vi "ReadDataByIdentifier.vi"(5 "LogSuspend":bool, 8 "error in":errorcluster, 10 "DID":string="02 02", 11 "UdsHandleIn":T1={"LogPath"=path "", "LogEnabled"=FALSE, "isOpen"=FALSE, "LogContent"="", "Adapter"="CAN0", "MCanHandle"={"MCanAdapter"=refnum}, "TransmittId"=0, "ReceiveId"=0}) -> (0 "error out":errorcluster, 2 "DataOut":string, 3 "UdsHandleOut":T1={"LogPath"=path "", "LogEnabled"=FALSE, "isOpen"=FALSE, "LogContent"="", "Adapter"="CAN0", "MCanHandle"={"MCanAdapter"=refnum}, "TransmittId"=0, "ReceiveId"=0})   [LabVIEW 2011, in "Konvolucio MUDS150628.lvlib"]
uses:
  <instrlib>/Konvolucio MUDS150628/Konvolucio MUDS150628.lvlib
  <instrlib>/Konvolucio MUDS150628/Types/UdsHandleType.ctl
  <instrlib>/Konvolucio MCAN120803/Types/MCanHandleType.ctl
  C:/Program Files/National Instruments/LabVIEW 2011/instr.lib/Konvolucio MCAN120803/Private/Konvolucio.MCAN120803.dll
  Konvolucio MCAN120803/Private/Konvolucio.MCAN120803.dll
  <instrlib>/Konvolucio MCAN120803/Konvolucio MCAN120803.lvlib
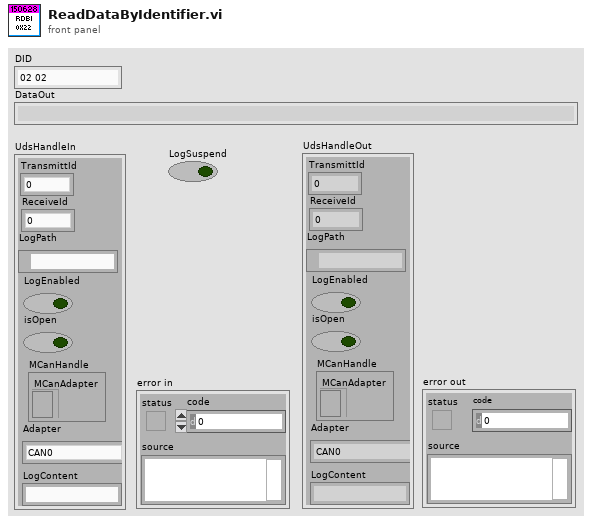
[diagram p1: front panel]
types:
  T1 = typedef "Konvolucio MUDS150628.lvlib/UdsHandleType.ctl" = cluster{"LogPath":path, "LogEnabled":bool, "isOpen":bool, "LogContent":string, "Adapter":string, "MCanHandle":T2, "TransmittId":u32, "ReceiveId":u32}
  T2 = typedef "Konvolucio MCAN120803.lvlib/MCanHandleType.ctl" = cluster{"MCanAdapter":refnum<k24>}
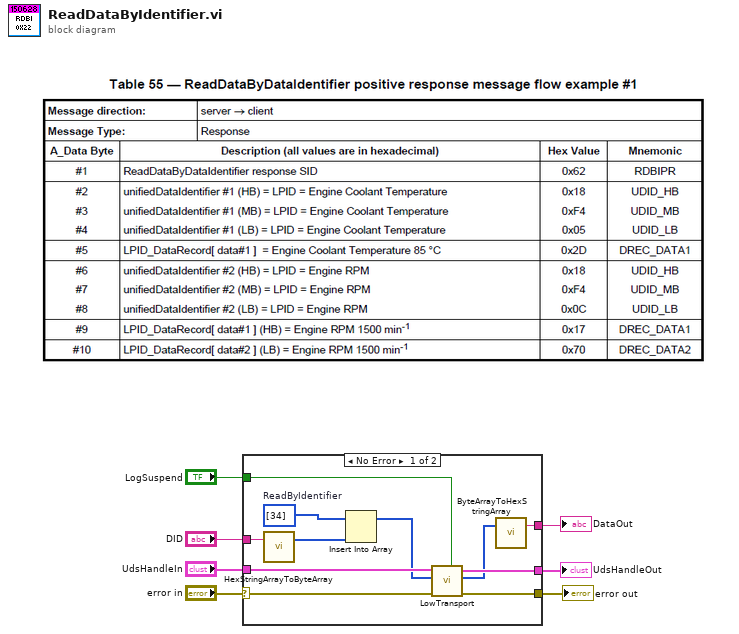
[diagram p0: block diagram]
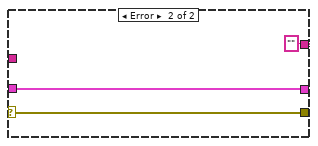
[diagram p2: hidden frame]
diagram:
  n1 = case shown="No Error" "error in" {
    selector: "error in" -> [w17 w21]
    tunnel: "UdsHandleIn" -> [w18 w20]
    tunnel: [w16 w21] -> w5
    tunnel: [w15 w20] -> w4
    tunnel: "LogSuspend" -> [w14 _]
    tunnel: [w11 "" ("trimmed string")] -> w2
    tunnel: "DID" -> [w8 _]
    frame No Error {
      w13 = u8[] [34]  # ReadByIdentifier
      n2 = call <instrlib>:"HexStringArrayToByteArray.vi"("HexStirngArray"=w8) -> ("ByteArrayOut"=w9:u8[])  [unwired: 2 in]
      n3 = Insert Into Array(array=w13, new element=w9) -> (w12:u8[])  [unwired: 1 in]
      n4 = call <instrlib>:"LowTransport.vi"("LogSuspend"=w14, "error in"=w17, "Request"=w12, "HandleIn"=w18) -> ("error out"=w16:errorcluster, "Response"=w10:u8[], "HandleOut"=w15:T1)  [unwired: 5 in]
      n5 = call <instrlib>:"ByteArrayToHexStringArray.vi"("ByteArrayIn"=w10) -> ("HexStringArrayOut"=w11:string)  [unwired: 2 in]
    }
    frame Error {
    }
  }
  "error out" <- w5
  "UdsHandleOut" <- w4
  "DataOut" <- w2
